vi "EJERCICIO 3 DE LOGICA COMBINACIONAL.vi"() -> ()   [LabVIEW 2013]
panel:
  out "Boolean 4":bool
  in  "Z":bool
  in  "Y":bool
  in  "X":bool
  # "universidad de cundinamarca \ningenieria de sistemas \nandy leandro camargo\nelectiva pro IV"
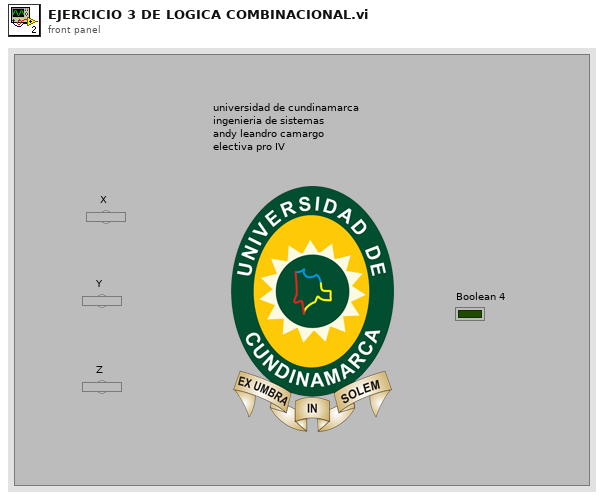
[diagram p1: front panel]
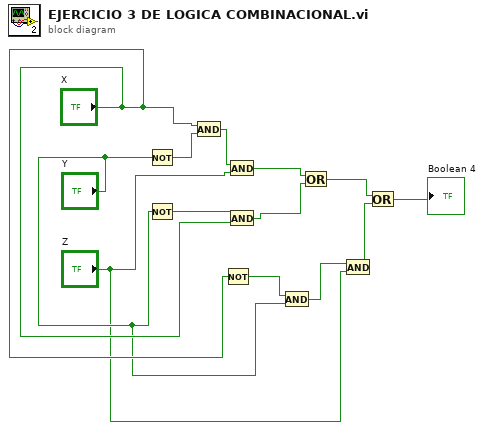
[diagram p0: block diagram]
diagram:
  n1 = Not(x="Y") -> (.not. x?=w13:bool)
  n2 = Not(x="Y") -> (.not. x?=w10:bool)
  n3 = And(x="X", y=w13) -> (x .and. y?=w12:bool)
  n4 = Not(x="X") -> (.not. x?=w7:bool)
  n5 = And(x=w12, y="Z") -> (x .and. y?=w11:bool)
  n6 = And(x=w10, y="X") -> (x .and. y?=w9:bool)
  n7 = And(x=w7, y="Y") -> (x .and. y?=w6:bool)
  n8 = Or(x=w11, y=w9) -> (x .or. y?=w3:bool)
  n9 = And(x=w6, y="Z") -> (x .and. y?=w4:bool)
  n10 = Or(x=w3, y=w4) -> (x .or. y?=→"Boolean 4":bool)
